vi "Pop Up.vi"() -> (3 "Pop Up Msg out":refnum<class "Pop Up Msg.lvclass">)   [LabVIEW 2021, in "Pop Up.lvlib" / "Pop Up Msg.lvclass"]
uses:
  Pop Up Msg.lvclass
  Pop Up Msg.lvclass/Pop Up Msg.ctl
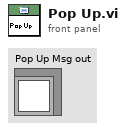
[diagram p1: front panel]
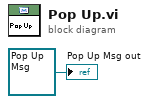
[diagram p0: block diagram]
diagram:
  "Pop Up Msg out" <- refnum<class "Pop Up Msg.lvclass"> refnum ("Pop Up Msg Strategy out")
